vi "Get Ctl Refs Within DVR.vi"(8 "error in (no error)":errorcluster, 10 "DVR Ref":refnum<vi>) -> (0 "error out":errorcluster, 2 "Controls[]":refnum<vi>[](array[refnum]))   [LabVIEW 2018, in "DVR Accessor Library.lvlib"]
uses:
  <vilib>/Utility/traverseref.llb/TRef TravTarget.ctl
  DVR Accessor Library.lvlib
  <vilib>/Utility/traverseref.llb/VI Scripting - Traverse.lvlib
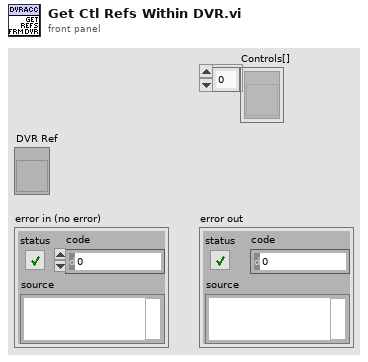
[diagram p1: front panel]
types:
  T1 = typedef "TRef TravTarget.ctl" = enum16{"FP", "BD", "Other"}
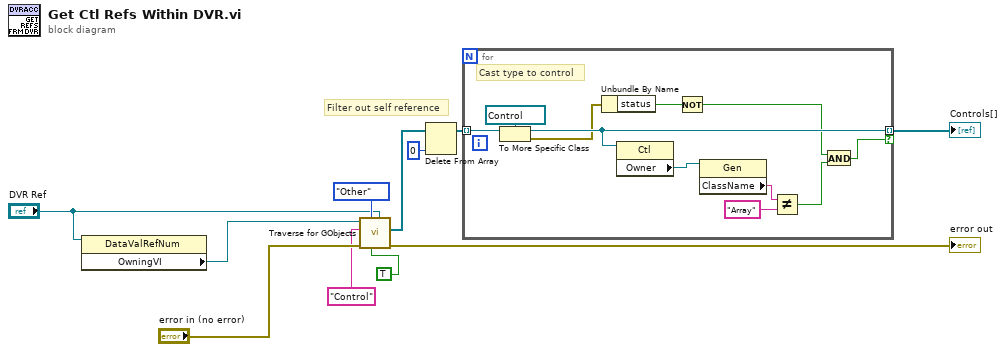
[diagram p0: block diagram]
diagram:
  # "Filter out self reference"
  n1 = property on="Property Node" class="DataValRefNum"(reference="DVR Ref") -> ("OwningVI"=w2:refnum<vi>)  [unwired: 1 in, 2 out]
  n2 = call <vilib>:"Traverse for GObjects.vi"("Other Refnum"="DVR Ref", "Traverse Generated Code (F)"=TRUE, "Traverse Target"=TRef_TravTarget."Other", "error in (no error)"="error in (no error)", "Class Name"="Control", "VI Refnum"=w2) -> ("error out"=→"error out":errorcluster, "References"=w8:refnum<vi>[])  [unwired: 2 in, 2 out]
  n3 = Delete From Array(array=w8, index=0) -> (array with subset deleted=w10:refnum<vi>[])  [unwired: 1 in, 1 out]
  n4 = for {
    tunnel: w10 -> [w22] mode=indexing
    tunnel: [w17] -> w11 mode=indexing if=w12
    # "Cast type to control"
    n5 = To More Specific Class(target class=refnum<vi> refnum ("Source Object Reference"), reference=w22) -> (specific class reference=w17:refnum<vi>, error out=w16:errorcluster)  [unwired: 1 in]
    n6 = Unbundle By Name(w16) -> ("status"=w15:bool)
    n7 = property class="Ctl"(reference=w17) -> ("Owner"=w20:refnum<vi>)  [unwired: 1 in, 2 out]
    n8 = Not(x=w15) -> (.not. x?=w13:bool)
    n9 = property class="Gen"(reference=w20) -> ("ClassName"=w19:string)  [unwired: 1 in, 2 out]
    n10 = Not Equal?(x=w19, y="Array") -> (x != y?=w14:bool)
    n11 = And(x=w13, y=w14) -> (x .and. y?=w12:bool)
  }
  "Controls[]" <- w11
